vi "robot ver2.vi"() -> ()   [LabVIEW 2021]
uses:
  <vilib>/userDefined/High Color/IMAQdx.ctl
  <vilib>/vision/Pattern Matching.llb/IMAQ Curve Parameters.ctl
  <vilib>/vision/driver/IMAQdx.llb/IMAQdx Buffer Number Mode.ctl
  <vilib>/vision/driver/NI_Vision_Acquisition_Software.lvlib
  <vilib>/vision/NI_Vision_Development_Module.lvlib
panel:
  in  "address ip":string
  in  "Stop Button":bool
  in  "Learn":bool
  out "Template":T1(plugin-control)
  in  "Curve Parameters":T2={"Extraction Mode"=0, "Edge Threshold"=75, "Edge Filter Size"=1, "Min Length"=25, "Row Search Step Size"=15, "Col Search Step Size"=15, "Max Endpoint Gap"=10, "Closed"=FALSE, "Subpixel"=FALSE} {"Max Endpoint Gap" min=0; "Col Search Step Size" min=1 max=255 step=1; "Row Search Step Size" min=1 max=255 step=1; "Min Length" min=0; "Edge Filter Size" items=["Fine", "Normal", "Controur Tracing"]; "Edge Threshold" min=1 max=65535 step=1; "Extraction Mode" items=["Normal", "Uniform Regions"]}
  in  "Snap Frame":bool
  out "Snap Image":T1(plugin-control)
  in  "Camera Name":T3="cam0"
  out "Image Out":T1(plugin-control)
  in  "Match":bool
  in  "Minimum Contrast":i32=10
  in  "Pattern Match Mode":u16(ring) items=["Shift Invariant", "Rotation Invariant"]
  out "Matches":T4(array[cluster]) {"Bounding Box"."y" format="%.2f"; "Bounding Box"."x" format="%.2f"; "Position"."y" format="%.2f"; "Position"."x" format="%.2f"; "Score" format="%.2f"; "Scale" format="%.2f"; "Angle" format="%.2f"}
  in  "Geometric Match Mode":T5={"Rotation"=TRUE, "Scale"=FALSE, "Occlusion"=FALSE, "Reserved"=FALSE, "Reserved"=FALSE, "Reserved"=FALSE}
  in  "Number of Matches":i32=1
  in  "Minimum Score":sgl=600.0
  in  "Subpixel Accuracy":bool
  in  "Match Type":enum16{"Geometric Matching", "Pattern Matching"}(ring)=enum."Pattern Matching"
  in  "Process Stop Button 3":bool
  in  "?":bool
  in  "speech to speech":bool
  in  "Object-Avoidance-System auto":bool
  in  "Object-Avoidance-System manuel":bool
  in  "avance 2":bool
  in  "reculer 2":bool
  in  "Gauche 2":bool
  in  "droite 2":bool
  in  "Stop  2":bool
  in  "data to send":string
  # "robot rocky"
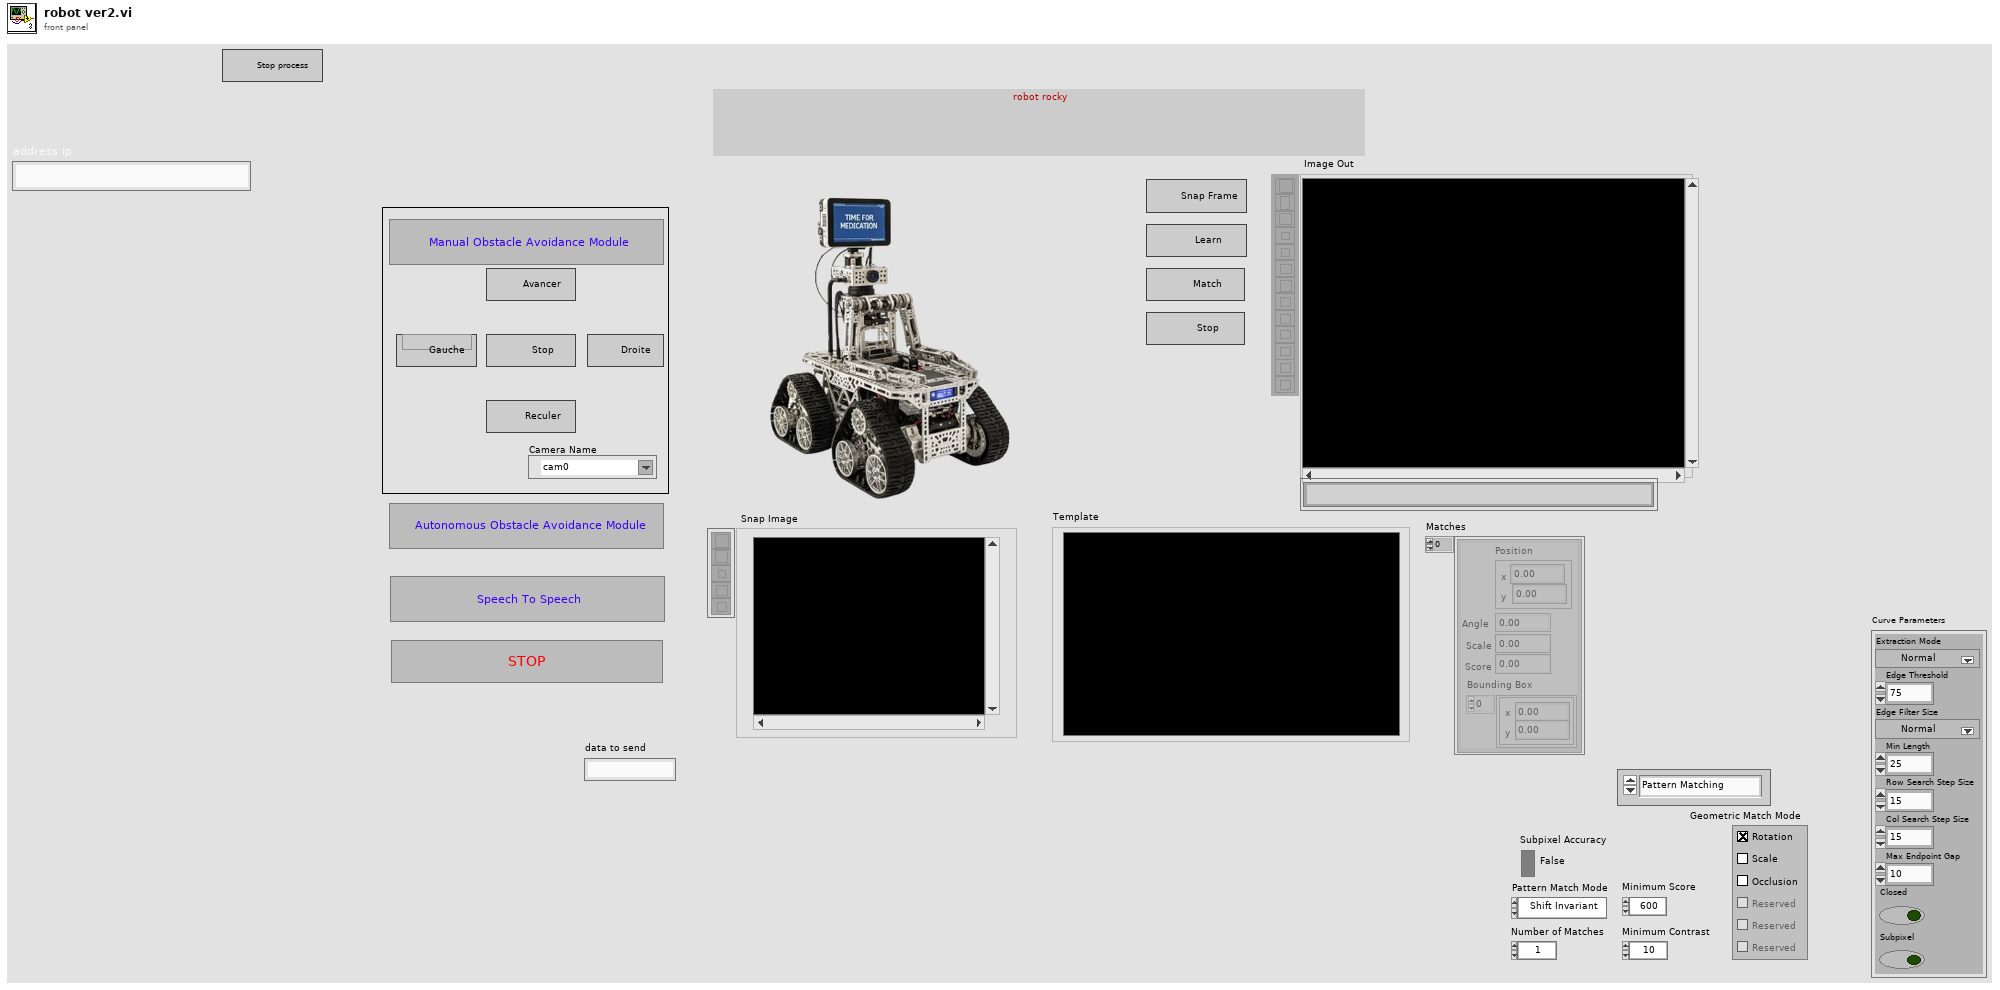
[diagram p1: front panel]
types:
  T1 = typedef "IMAQ Image.ctl" = refnum<image>
  T2 = typedef "IMAQ Curve Parameters.ctl" = cluster{"Extraction Mode":u32, "Edge Threshold":i32, "Edge Filter Size":u32, "Min Length":i32, "Row Search Step Size":i32, "Col Search Step Size":i32, "Max Endpoint Gap":i32, "Closed":bool, "Subpixel":bool}
  T3 = typedef "IMAQdx.ctl" = refnum<k21>
  T4 = cluster{"Position":cluster{"x":sgl, "y":sgl}, "Angle":sgl, "Scale":sgl, "Score":sgl, "Bounding Box":cluster{"x":sgl, "y":sgl}[]}[]
  T5 = cluster{"Rotation":bool, "Scale":bool, "Occlusion":bool, "Reserved":bool, "Reserved":bool, "Reserved":bool}
  T6 = cluster{"Global Rectangle":i32[], "Contours":cluster{"Contour Type":u32, "ROI Type":u32, "Points":i32[]}[]}
  T7 = typedef "NI_Vision_Acquisition_Software.lvlib/IMAQdx Buffer Number Mode.ctl" = enum32{"Next", "Last", "Buffer Number", "Every", "Last New"}
  T8 = cluster{i32[], cluster{"Contour Type":u32, "ROI Type":u32, i32[]}[]}
  T9 = typedef "Image Type" = u32
  T10 = typedef "IMAQ GM Match Report.ctl" = cluster{"Position":cluster{"x":sgl, "y":sgl}, "Angle":sgl, "Scale":sgl, "Score":sgl, "Bounding Box":cluster{"x":sgl, "y":sgl}[], "Contrast Reversed":bool, "Occlusion %":sgl, "Template Target Curve Score":sgl, "Target Template Curve Score":sgl, "Correlation Score":sgl}
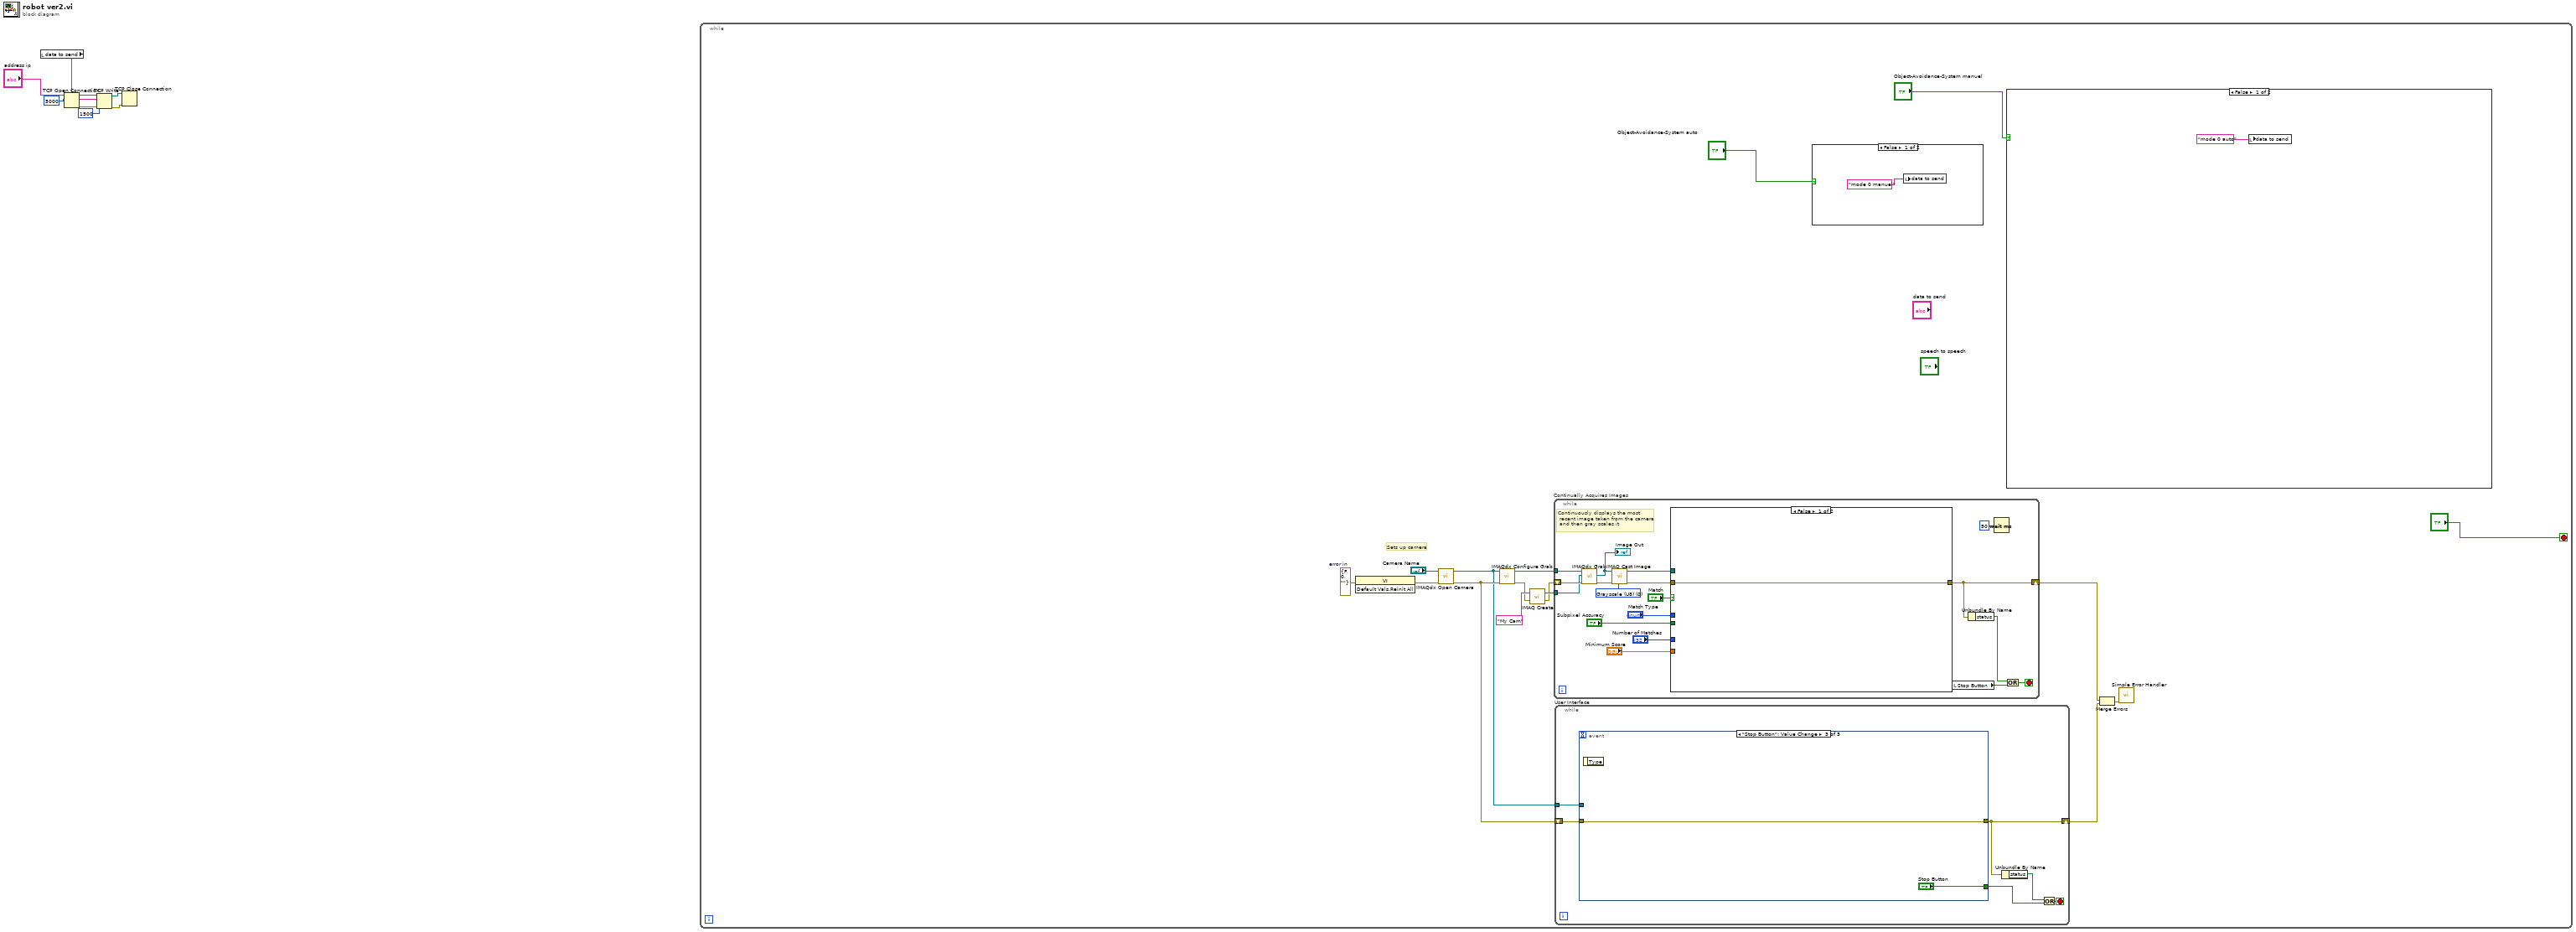
[diagram p0: block diagram]
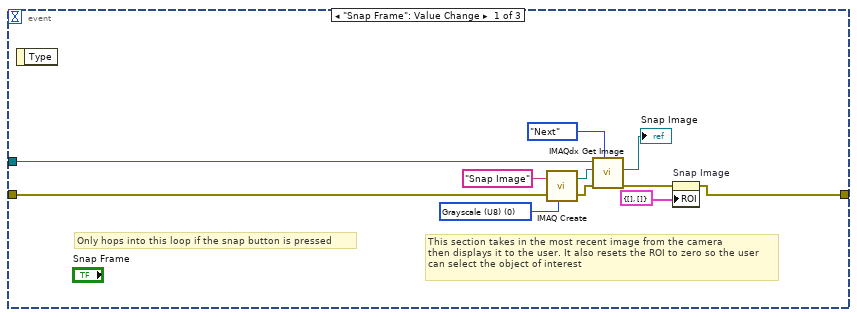
[diagram p2: hidden frame]
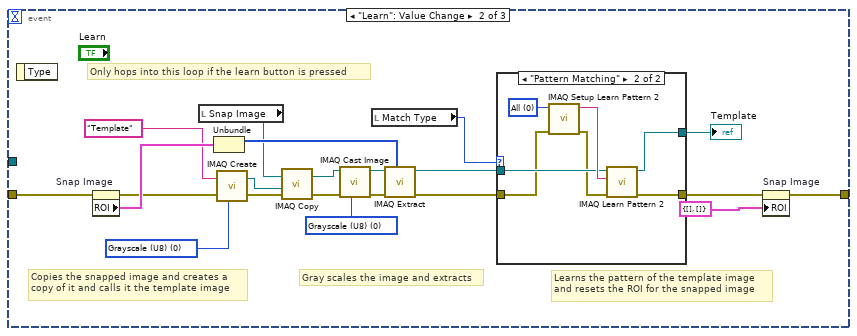
[diagram p3: hidden frame]
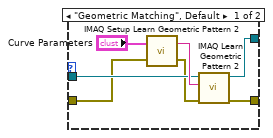
[diagram p4: hidden frame]
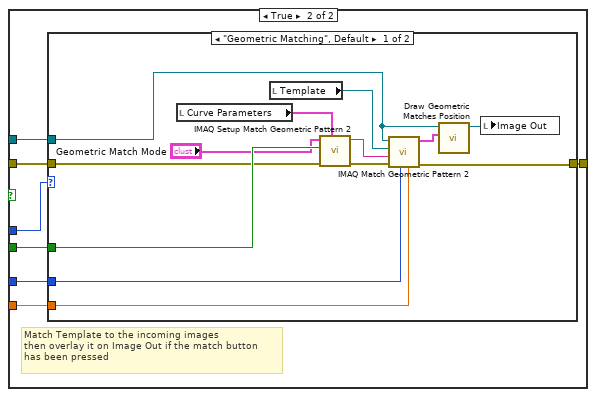
[diagram p5: hidden frame]
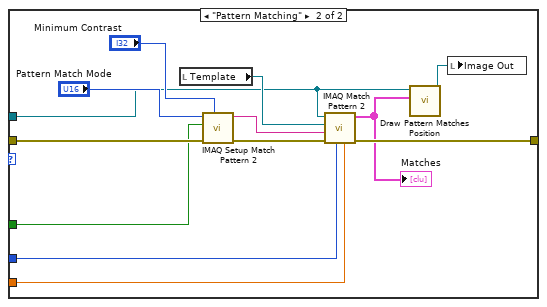
[diagram p6: hidden frame]
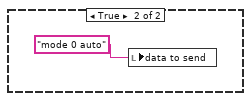
[diagram p7: hidden frame]
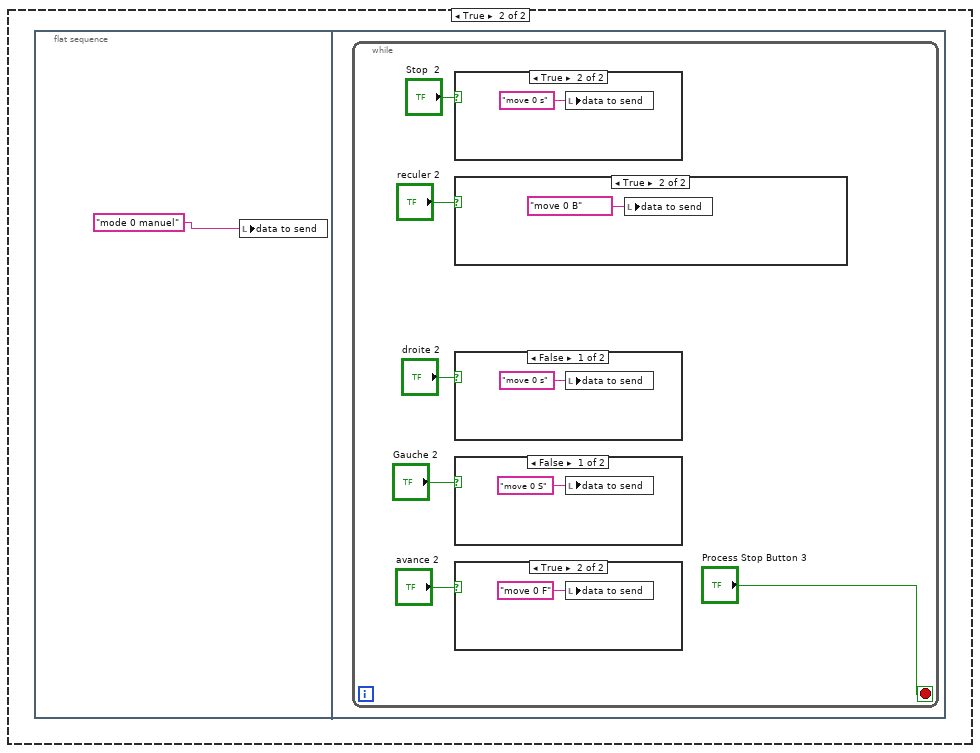
[diagram p8: hidden frame]
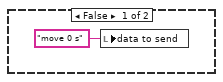
[diagram p9: hidden frame]
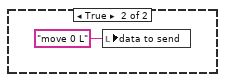
[diagram p10: hidden frame]
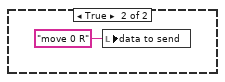
[diagram p11: hidden frame]
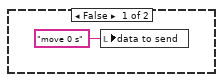
[diagram p12: hidden frame]
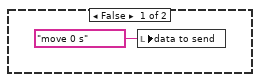
[diagram p13: hidden frame]
diagram:
  n1 = local read "data to send"() -> (w7:string)
  n2 = TCP Open Connection(address="address ip", remote port or service name=u16 5000) -> (connection ID=w6:refnum<k5>, error out=w8:errorcluster)  [unwired: 3 in]
  n3 = TCP Write(connection ID=w6, data in=w7, error in (no error)=w8, 9:1500 ("timeout ms (25000)")) -> (connection ID out=w3:refnum<k5>, error out=w4:errorcluster)  [unwired: 1 out]
  n4 = TCP Close Connection(connection ID=w3, error in (no error)=w4) -> ()  [unwired: 1 in, 2 out]
  n5 = while {
    stop <- "?" stop-if-true
    w19 = errorcluster {"status"=FALSE, "code"=0, "source"=""}  # error in
    # "Sets up camera"
    n6 = invoke class="VI" method="Default Vals.Reinit All"(error in=w19) -> (error out=w18:errorcluster)  [unwired: 2 in, 2 out]
    n7 = call <vilib>:"IMAQdx Open Camera.vi"("error in"=w18, "Session In"="Camera Name") -> ("error out"=w15:errorcluster, "Session Out"=w14:T3)  [unwired: 8 in]
    n8 = call <vilib>:"IMAQdx Configure Grab.vi"("error in"=w15, "Session In"=w14) -> ("error out"=w10:errorcluster, "Session Out"=w21:T3)  [unwired: 8 in]
    n9 = call "IMAQ Create"("Image Name"="My Cam", "error in (no error)"=w10) -> ("New Image"=w17:T1, "error out"=w9:errorcluster)  [unwired: 3 in]
    n10 = while "Continually Acquires Images" {
      tunnel: w21 -> [w96]
      tunnel: w17 -> [w94]
      shift-right: [w86] -> w12
      shift-left: w9 -> [w95]
      stop <- w87 stop-if-true
      w91 = T9 0 items=["Grayscale (U8)", "Grayscale (I16)", "Grayscale (SGL)", "Complex (CSG)", "RGB (U32)", "HSL (U32)", "RGB (U64)", "Grayscale (U16)"] ("Image Type")
      # "Continuously displays the most\n recent image taken from the camera\n and then gray scales it"
      n11 = call <vilib>:"IMAQdx Grab.vi"("error in"=w95, "Image In"=w94, "Session In"=w96) -> ("error out"=w92:errorcluster, "Image Out"=w93:T1)  [unwired: 5 in, 2 out]
      "Image Out" <- w93
      n12 = call "IMAQ Cast Image"("Image Type"=w91, "error in (no error)"=w92, "Image Src"=w93) -> ("error out"=w80:errorcluster, "Image Dst Out"=w90:T1)  [unwired: 7 in]
      n13 = case shown="False" "Match" {
        tunnel: w80 -> [w97 w98]
        tunnel: w90 -> [_ w104]
        tunnel: [w97 w103] -> w86
        tunnel: "Number of Matches" -> [_ w102]
        tunnel: "Minimum Score" -> [_ w101]
        tunnel: "Subpixel Accuracy" -> [_ w100]
        tunnel: "Match Type" -> [_ w99]
        frame False {
        }
        frame True {
          # "Match Template to the incoming images \nthen overlay it on Image Out if the match button\nhas been pressed"
          n14 = case shown="\"Geometric Matching\", Default" w99 {
            tunnel: w98 -> [w107 w125]
            tunnel: w104 -> [w110 w119]
            tunnel: [w114 w124] -> w103
            tunnel: w102 -> [w112 w123]
            tunnel: w101 -> [w111 w122]
            tunnel: w100 -> [w109 w121]
            frame "Geometric Matching", Default {
              n15 = local read "Curve Parameters"() -> (w116:T2)
              n16 = local read "Template"() -> (w117:T1)
              n17 = call "IMAQ Setup Match Geometric Pattern 2"("Curve Parameters"=w116, "error in (no error)"=w107, "Subpixel Accuracy"=w109, "Match Mode"="Geometric Match Mode") -> ("error out"=w105:errorcluster, "Match Geometric Pattern 2 Setup Data"=w115:string)  [unwired: 6 in]
              n18 = call "IMAQ Match Geometric Pattern 2"("Minimum Match Score"=w111, "Number of Matches Requested"=w112, "error in (no error)"=w105, "Match Geometric Pattern 2 Setup Data"=w115, "Template Image"=w117, "Image"=w110) -> ("error out"=w114:errorcluster, "Matches (pixel)"=w108:T10[])  [unwired: 2 in, 2 out]
              n19 = call "Draw Geometric Matches Position .vi"("Matches (pixel)"=w108, "Image"=w110) -> ("Image Out"=w113:T1)  [unwired: 9 in]
              n20 = local write "Image Out"(w113) -> ()
            }
            frame "Pattern Matching" {
              n21 = local read "Template"() -> (w127:T1)
              n22 = call "IMAQ Setup Match Pattern 2"("Minimum Contrast"="Minimum Contrast", "error in (no error)"=w125, "Subpixel Accuracy"=w121, "Match Mode"="Pattern Match Mode") -> ("error out"=w126:errorcluster, "Match Pattern Setup Data"=w130:string)  [unwired: 1 in, 5 out]
              n23 = call "IMAQ Match Pattern 2"("Minimum Match Score"=w122, "Number of Matches Requested"=w123, "error in (no error)"=w126, "Match Pattern Setup Data"=w130, "Template Image"=w127, "Image"=w119) -> ("error out"=w124:errorcluster, "Matches"=w120:T4)  [unwired: 1 in, 3 out]
              "Matches" <- w120
              n24 = call "Draw Pattern Matches Position .vi"("Matches"=w120, "Image"=w119) -> ("Image Out"=w118:T1)  [unwired: 9 in]
              n25 = local write "Image Out"(w118) -> ()
            }
          }
        }
      }
      n26 = local read "Stop Button"() -> (w88:bool)
      n27 = Unbundle By Name(w86) -> ("status"=w85:bool)
      n28 = Wait (ms)(milliseconds to wait=u32 50) -> ()  [unwired: 1 out]
      n29 = Or(x=w85, y=w88) -> (x .or. y?=w87:bool)
    }
    n30 = while "User Interface" {
      tunnel: w14 -> [w29]
      shift-right: [w26] -> w11
      shift-left: w15 -> [w30]
      stop <- w28 stop-if-true
      n31 = event shown="[2] \"Stop Button\": Value Change" {
        selector: _ -> [_ _ _]
        dyn-events: _ -> [_ _ _]
        timeout: _ -> [_ _ _]
        tunnel: [_ _ "Stop Button"] -> w27
        tunnel: w30 -> [w36 w60 w77]
        tunnel: w29 -> [w35 _ _]
        tunnel: [w31 w56 w77] -> w26
        event "Snap Frame": Value Change {
          w34 = T9 0 items=["Grayscale (U8)", "Grayscale (I16)", "Grayscale (SGL)", "Complex (CSG)", "RGB (U32)", "HSL (U32)", "RGB (U64)", "Grayscale (U16)"] ("Image Type")
          # "Only hops into this loop if the snap button is pressed"
          # "This section takes in the most recent image from the camera \nthen displays it to the user. It also resets the ROI to zero so the user\ncan select the object of interest"
          n32 = event-data() -> ()  [unwired: 1 in, 1 out]
          n33 = call "IMAQ Create"("Image Name"="Snap Image", "Image Type"=w34, "error in (no error)"=w36) -> ("New Image"=w39:T1, "error out"=w38:errorcluster)  [unwired: 2 in]
          n34 = call <vilib>:"IMAQdx Get Image.vi"("Buffer Number Mode (Next)"=IMAQdx_Buffer_Number_Mode."Next", "error in"=w38, "Image In"=w39, "Session In"=w35) -> ("error out"=w33:errorcluster, "Image Out"=→"Snap Image":T1)  [unwired: 4 in, 2 out]
          n35 = property on="Snap Image" class="ImageControl"(error in=w33, "ROI"=T6 {"Global Rectangle"=[], "Contours"=[]}) -> (error out=w31:errorcluster)  [unwired: 1 in, 1 out]
        }
        event "Learn": Value Change {
          w51 = T9 0 items=["Grayscale (U8)", "Grayscale (I16)", "Grayscale (SGL)", "Complex (CSG)", "RGB (U32)", "HSL (U32)", "RGB (U64)", "Grayscale (U16)"] ("Image Type")
          w52 = T9 0 items=["Grayscale (U8)", "Grayscale (I16)", "Grayscale (SGL)", "Complex (CSG)", "RGB (U32)", "HSL (U32)", "RGB (U64)", "Grayscale (U16)"] ("Image Type")
          # "Learns the pattern of the template image\nand resets the ROI for the snapped image"
          # "Gray scales the image and extracts"
          # "Copies the snapped image and creates a \ncopy of it and calls it the template image"
          # "Only hops into this loop if the learn button is pressed"
          n36 = event-data() -> ()  [unwired: 1 in, 1 out]
          n37 = property on="Snap Image" class="ImageControl"(error in=w60) -> (error out=w44:errorcluster, "ROI"=w59:T6)  [unwired: 1 in, 1 out]
          n38 = local read "Snap Image"() -> (w54:T1)
          n39 = Unbundle(w59) -> ("Global Rectangle"=w58:i32[])  [unwired: 1 out]
          n40 = call "IMAQ Create"("Image Name"="Template", "Image Type"=w52, "error in (no error)"=w44) -> ("New Image"=w42:T1, "error out"=w43:errorcluster)  [unwired: 2 in]
          n41 = call "IMAQ Copy"("error in (no error)"=w43, "Image Dst"=w42, "Image Src"=w54) -> ("error out"=w48:errorcluster, "Image Dst Out"=w50:T1)  [unwired: 3 in]
          n42 = call "IMAQ Cast Image"("Image Type"=w51, "error in (no error)"=w48, "Image Src"=w50) -> ("error out"=w47:errorcluster, "Image Dst Out"=w49:T1)  [unwired: 7 in]
          n43 = local read "Match Type"() -> (w46:enum16{"Geometric Matching", "Pattern Matching"})
          n44 = call "IMAQ Extract"("Optional Rectangle"=w58, "error in (no error)"=w47, "Image Src"=w49) -> ("error out"=w45:errorcluster, "Image Dst Out"=w62:T1)  [unwired: 3 in, 4 out]
          n45 = case shown="\"Pattern Matching\"" w46 {
            tunnel: w62 -> [w65 w75]
            tunnel: [w66 w73] -> w61
            tunnel: [w67 w71] -> w57
            tunnel: w45 -> [w64 w70]
            frame "Geometric Matching", Default {
              n46 = call "IMAQ Setup Learn Geometric Pattern 2"("error in (no error)"=w64, "Curve Parameters"="Curve Parameters") -> ("error out"=w63:errorcluster, "Learn Geometric Pattern 2 Setup Data"=w68:string)
              n47 = call "IMAQ Learn Geometric Pattern 2"("error in (no error)"=w63, "Learn Geometric Pattern 2 Setup Data"=w68, "Template Image"=w65) -> ("error out"=w67:errorcluster, "Template Image Out"=w66:T1)  [unwired: 7 in]
            }
            frame "Pattern Matching" {
              w74 = u16 0 items=["All", "Shift Information", "Rotation Information"] ("Learn Mode")
              n48 = call "IMAQ Setup Learn Pattern 2"("error in (no error)"=w70, "Learn Mode"=w74) -> ("error out"=w72:errorcluster, "Learn Pattern Setup Data"=w76:string)  [unwired: 8 out]
              n49 = call "IMAQ Learn Pattern 2"("error in (no error)"=w72, "Learn Pattern Setup Data"=w76, "Image"=w75) -> ("error out"=w71:errorcluster, "Template Image Out"=w73:T1)  [unwired: 1 in, 6 out]
            }
          }
          "Template" <- w61
          n50 = property on="Snap Image" class="ImageControl"(error in=w57, "ROI"=T8 {[], []}) -> (error out=w56:errorcluster)  [unwired: 1 in, 1 out]
        }
        event "Stop Button": Value Change {
          n51 = event-data() -> ()  [unwired: 1 in, 1 out]
        }
      }
      n52 = Unbundle By Name(w26) -> ("status"=w25:bool)
      n53 = Or(x=w25, y=w27) -> (x .or. y?=w28:bool)
    }
    n54 = case shown="False" "Object-Avoidance-System auto" {
      frame False {
        n55 = local write "data to send"("mode 0 manuel" ("write buffer")) -> ()
      }
      frame True {
        n56 = local write "data to send"("mode 0 auto" ("write buffer")) -> ()
      }
    }
    n57 = case shown="False" "Object-Avoidance-System manuel" {
      frame False {
        n58 = local write "data to send"("mode 0 auto" ("write buffer")) -> ()
      }
      frame True {
        n59 = flat-sequence {
          frame #0 {
            n60 = local write "data to send"("mode 0 manuel" ("write buffer")) -> ()
          }
          frame #1 {
            n61 = while {
              stop <- "Process Stop Button 3" stop-if-true
              n62 = case shown="True" "Stop  2" {
                frame False {
                  n63 = local write "data to send"("move 0 s" ("write buffer")) -> ()
                }
                frame True {
                  n64 = local write "data to send"("move 0 s") -> ()
                }
              }
              n65 = case shown="True" "reculer 2" {
                frame False {
                  n66 = local write "data to send"("move 0 s") -> ()
                }
                frame True {
                  n67 = local write "data to send"("move 0 B") -> ()
                }
              }
              n68 = case shown="False" "droite 2" {
                frame False {
                  n69 = local write "data to send"("move 0 s") -> ()
                }
                frame True {
                  n70 = local write "data to send"("move 0 R") -> ()
                }
              }
              n71 = case shown="False" "Gauche 2" {
                frame False {
                  n72 = local write "data to send"("move 0 S") -> ()
                }
                frame True {
                  n73 = local write "data to send"("move 0 L") -> ()
                }
              }
              n74 = case shown="True" "avance 2" {
                frame False {
                  n75 = local write "data to send"("move 0 s") -> ()
                }
                frame True {
                  n76 = local write "data to send"("move 0 F") -> ()
                }
              }
            }
          }
        }
      }
    }
    n77 = Merge Errors(w12, w11) -> (w13:errorcluster)
    n78 = call <vilib>:"Simple Error Handler.vi"("error in (no error)"=w13) -> ()  [unwired: 4 in, 5 out]
  }
